vi "for循环.vi"() -> ()   [LabVIEW 2017]
panel:
  out "波形图表":dbl(graph)
  out "数值 2":i32
  out "数值":dbl
  out "布尔":bool
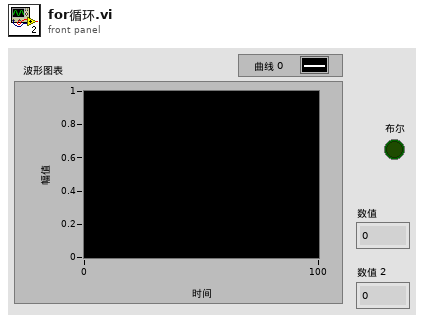
[diagram p1: front panel]
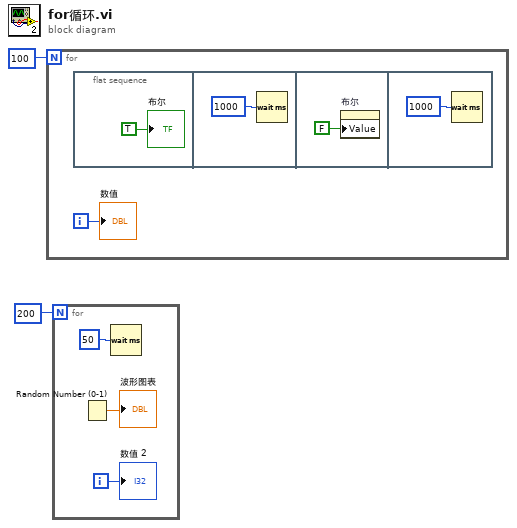
[diagram p0: block diagram]
diagram:
  n1 = for {
    N: 100 -> [_]
    i -> [w3]
    n2 = flat-sequence {
      frame #0 {
        "布尔" <- TRUE ("布尔")
      }
      frame #1 {
        n3 = Wait (ms)(milliseconds to wait=u32 1000 ("等待时间（毫秒）")) -> ()  [unwired: 1 out]
      }
      frame #2 {
        n4 = property on="布尔" class="Bool (严格)"("Value"=FALSE ("布尔")) -> ()  [unwired: 2 in, 2 out]
      }
      frame #3 {
        n5 = Wait (ms)(milliseconds to wait=u32 1000 ("等待时间（毫秒）")) -> ()  [unwired: 1 out]
      }
    }
    "数值" <- w3
  }
  n6 = for {
    N: 200 -> [_]
    i -> [w10]
    n7 = Random Number (0-1)() -> (number: 0 to 1=→"波形图表":dbl)
    n8 = Wait (ms)(milliseconds to wait=u32 50 ("等待时间（毫秒）")) -> ()  [unwired: 1 out]
    "数值 2" <- w10
  }
